vi "Check if string can be used as filename.vi"(1 "String with ext.":string) -> (0 "can be filename?":bool)   [LabVIEW 2009, in "FileIO lib.lvlib"]
doc: "Checks to see if input string could be used for filename stub (no extension)."
uses:
  FileIO lib.lvlib
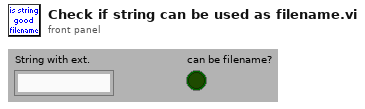
[diagram p1: front panel]
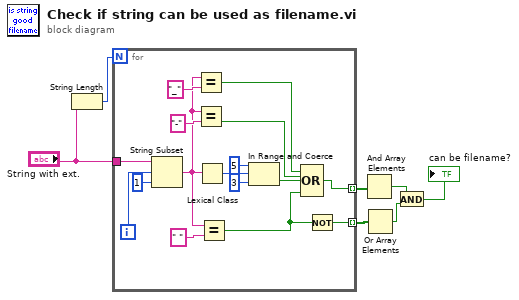
[diagram p0: block diagram]
diagram:
  n1 = String Length(string="String with ext.") -> (length=w6:i32)
  n2 = for {
    N: w6 -> [_]
    tunnel: "String with ext." -> [w23]
    tunnel: [w16] -> w5 mode=indexing
    tunnel: [w15] -> w3 mode=indexing
    i -> [w17]
    n3 = String Subset(string=w23, offset (0)=w17, length (rest)=1 ("length (rest)")) -> (substring=w8:string)
    n4 = Equal?(x=w8, y="_") -> (x = y?=w10:bool)
    n5 = Equal?(x=w8, y="-") -> (x = y?=w9:bool)
    n6 = Lexical Class(1:w8) -> (0:w21:i16)
    n7 = Equal?(x=w8, y=" ") -> (x = y?=w13:bool)
    n8 = In Range and Coerce(upper limit=i16 5, x=w21, lower limit=i16 3) -> (In Range?=w18:bool)  [unwired: 1 out]
    n9 = Compound Arithmetic op=OR(w10, w9, w18, w13) -> (w15:bool)
    n10 = Not(x=w13) -> (.not. x?=w16:bool)
  }
  n11 = And Array Elements(Boolean array=w3) -> (logical AND=w2:bool)
  n12 = Or Array Elements(Boolean array=w5) -> (logical OR=w4:bool)
  n13 = And(x=w2, y=w4) -> (x .and. y?=→"can be filename?":bool)
